vi "OSF Create Projects.vi"(8 "error in":errorcluster, 9 "Proposal Data":T1, 10 "Token":string="https://api.osf.io/v2/", 11 "OSF API URL":string="https://api.osf.io/v2/") -> (0 "error out":errorcluster, 2 "Wiki ID":string)   [LabVIEW 2020]
uses:
  Utilities/iCalendar/Extract iCalendar String.ctl
  <vilib>/httpClient/POSTBuffer.vi
  <vilib>/httpClient/LabVIEWHTTPClient.lvlib
  <vilib>/JDP Science/JSONtext/JSONtext.lvlib
panel:
  in  "Wiki name":string="home"
  in  "Parse from":enum16{"Proposal HTML:", "Proposal cluster"}(ring)=enum."Proposal cluster"
  out "Create proj reply":string
  out "headers":string
  in  "Proposal document":path=path "C:/Users/l121767/Dropbox/Projects/FAIR/Project files/Proposal/National High Magnetic Field Laboratory - Users Program.html"
  out "body":string
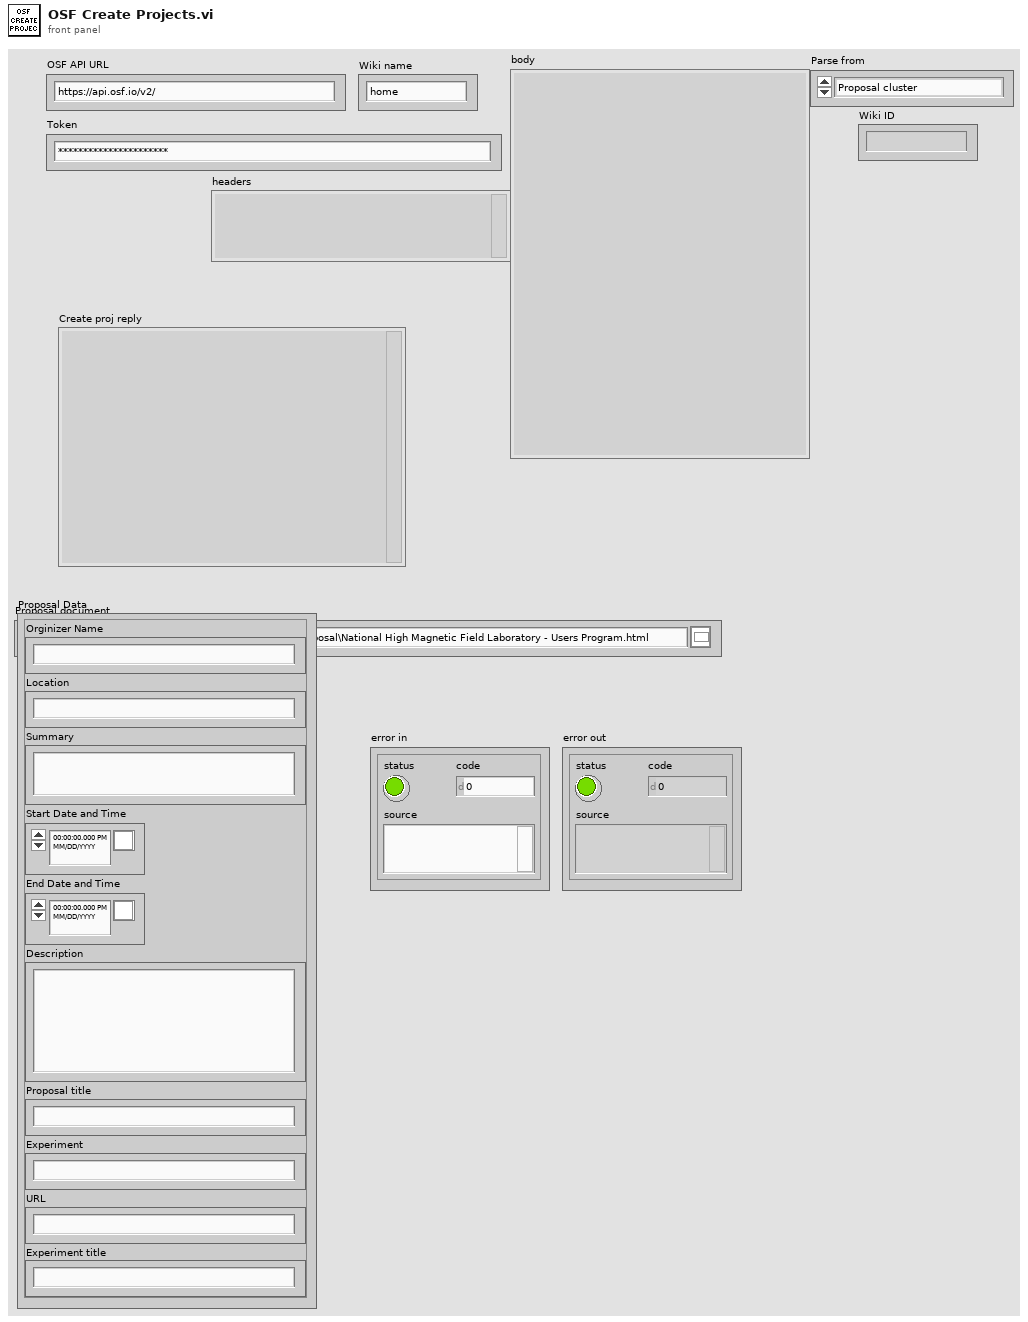
[diagram p1: front panel]
types:
  T1 = typedef "Extract iCalendar String.ctl" = cluster{"Orginizer Name":string, "Location":string, "Summary":string, "Start Date and Time":timestamp, "End Date and Time":timestamp, "Description":string, "Proposal title":string, "Experiment":string, "URL":string, "Experiment title":string}
  T2 = typedef "LabVIEWHTTPClient.lvlib/ClientHandle.ctl" = refnum<k1>
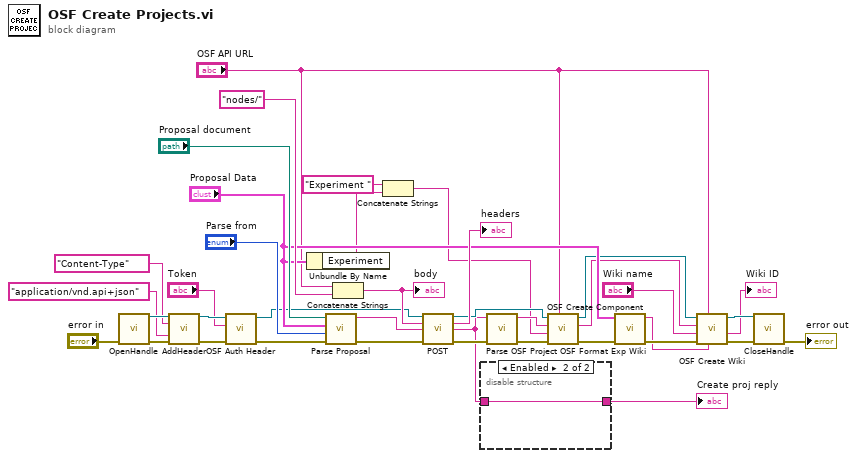
[diagram p0: block diagram]
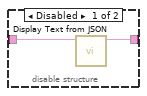
[diagram p2: hidden frame]
diagram:
  n1 = call <vilib>:"OpenHandle.vi"("error in (no error)"="error in") -> ("client handle out"=w37:T2, "error out"=w36:errorcluster)  [unwired: 13 in]
  n2 = call <vilib>:"AddHeader.vi"("client handle"=w37, "header"="Content-Type", "value"="application/vnd.api+json", "error in (no error)"=w36) -> ("client handle out"=w8:T2, "error out"=w6:errorcluster)  [unwired: 10 in]
  n3 = call "OSF Auth Header.vi"("error in"=w6, "Token"="Token", "client handle"=w8) -> ("error out"=w5:errorcluster, "client handle out"=w4:T2)  [unwired: 7 in]
  n4 = Unbundle By Name("Proposal Data") -> ("Experiment"=w2:string)
  n5 = call "Parse Proposal.vi"("error in"=w5, "Parse from"="Parse from", "Proposal Data"="Proposal Data", "Proposal document"="Proposal document") -> ("error out"=w32:errorcluster, "Puject  JSON"=w31:string)  [unwired: 6 in]
  n6 = Concatenate Strings("OSF API URL", "nodes/") -> (w30:string)
  "body" <- w30
  n7 = Concatenate Strings("Experiment " ("string"), w2) -> (w3:string)
  n8 = call-poly <vilib>:"POST.vi"("client handle"=w4, "url"=w30, "buffer"=w31, "error in (no error)"=w32) -> ("client handle out"=w23:T2, "headers"=→"headers":string, "body"=w9:string, "error out"=w25:errorcluster)  [unwired: 8 in]
  n9 = disable-structure shown="Enabled" {
    disable-tunnel: [w40 w41] -> w10
    disable-tunnel: w9 -> [w39 w41]
    frame Disabled {
      n10 = call <vilib>:"Display Text from JSON.vi"("Input JSON"=w39) -> ("Display Text"=w40:string)  [unwired: 8 in, 2 out]
    }
    frame Enabled {
    }
  }
  "Create proj reply" <- w10
  n11 = call "Parse OSF Project.vi"("error in"=w25, "Project JSON"=w9) -> ("error out"=w24:errorcluster, "Project ID"=w22:string)  [unwired: 7 in, 1 out]
  n12 = call "OSF Create Component.vi"("OSF API URL"="OSF API URL", "error in"=w24, "Child name"=w3, "Parent  ID"=w22, "client handle"=w23) -> ("error out"=w21:errorcluster, "Component ID"=w17:string, "client handle out"=w18:T2)  [unwired: 4 in]
  n13 = call "OSF Format Exp Wiki.vi"("error in"=w21, "Proposal Data"="Proposal Data") -> ("error out"=w19:errorcluster, "resulting string"=w15:string)  [unwired: 8 in]
  n14 = call "OSF Create Wiki.vi"("content"=w15, "OSF API URL"="OSF API URL", "error in"=w19, "Wiki name"="Wiki name", "Parent  ID"=w17, "client handle"=w18) -> ("error out"=w13:errorcluster, "Wiki ID"=→"Wiki ID":string, "client handle out"=w12:T2)  [unwired: 2 in, 1 out]
  n15 = call <vilib>:"CloseHandle.vi"("client handle"=w12, "error in (no error)"=w13) -> ("error out"=→"error out":errorcluster)  [unwired: 13 in]
